vi "Teleop_Calc_Elevation.vi"(11 "Teleop Local Data in":T1) -> (3 "Teleop Local Data out":T1)   [LabVIEW 2016]
uses:
  Typedefs/typedef_cluster_Teleop Local Data.ctl
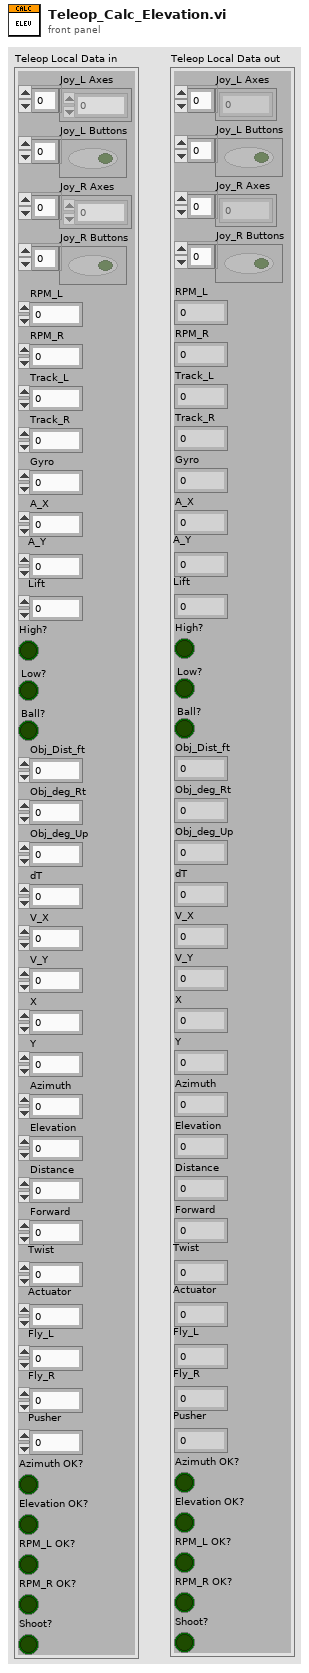
[diagram p1: front panel]
types:
  T1 = typedef "typedef_cluster_Teleop Local Data.ctl" = cluster{"Joy_L Axes":dbl[], "Joy_L Buttons":bool[], "Joy_R Axes":dbl[], "Joy_R Buttons":bool[], "RPM_L":dbl, "RPM_R":dbl, "Track_L":dbl, "Track_R":dbl, "Gyro":dbl, "A_X":dbl, "A_Y":dbl, "Lift":dbl, "High?":bool, "Low?":bool, "Ball?":bool, "Obj_Dist_ft":dbl, "Obj_deg_Rt":dbl, "Obj_deg_Up":dbl, "dT":dbl, "V_X":dbl, "V_Y":dbl, "X":dbl, "Y":dbl, "Azimuth":dbl, "Elevation":dbl, "Distance":dbl, "Forward":dbl, "Twist":dbl, "Actuator":dbl, "Fly_L":dbl, "Fly_R":dbl, "Pusher":dbl, "Azimuth OK?":bool, "Elevation OK?":bool, "RPM_L OK?":bool, "RPM_R OK?":bool, "Shoot?":bool}
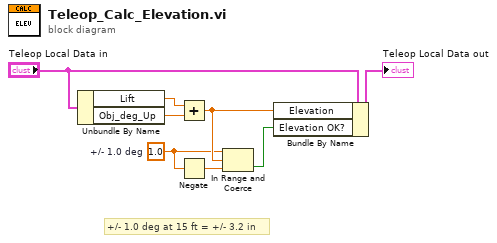
[diagram p0: block diagram]
diagram:
  w3 = 1.0  # +/- 1.0 deg
  # "+/- 1.0 deg at 15 ft = +/- 3.2 in"
  n1 = Unbundle By Name("Teleop Local Data in") -> ("Lift"=w5:dbl, "Obj_deg_Up"=w6:dbl)
  n2 = Add(x=w5, y=w6) -> (x+y=w4:dbl)
  n3 = Negate(x=w3) -> (-x=w2:dbl)
  n4 = In Range and Coerce(upper limit=w3, x=w4, lower limit=w2) -> (In Range?=w1:bool)  [unwired: 1 out]
  n5 = Bundle By Name(cluster="Teleop Local Data in", "Elevation"=w4, "Elevation OK?"=w1) -> (→"Teleop Local Data out":T1)
